vi "Parse Light IDs.vi"(8 "Error In":errorcluster, 10 "Light JSON":string="{\"1\":{\"name\": \"Hue Lamp\"},\"2\":{\"name\": \"Hue Lamp 1\"},\"3\":{\"name\": \"Hue Lamp 2\"}}") -> (0 "Error Out":errorcluster, 2 "Light IDs":i32[](array[numeric]))   [LabVIEW 2013, in "LMH-Hue.lvlib"]
uses:
  LMH-Hue.lvlib
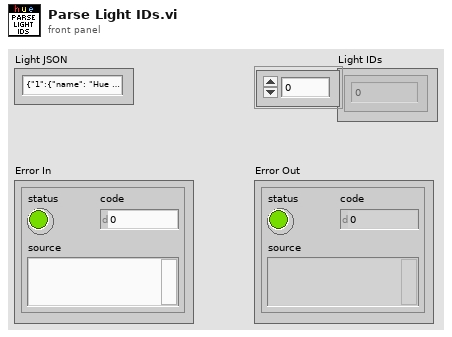
[diagram p1: front panel]
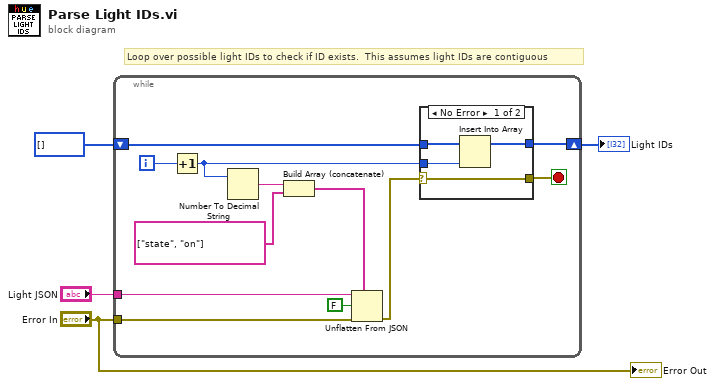
[diagram p0: block diagram]
diagram:
  # "Loop over possible light IDs to check if ID exists.  This assumes light IDs are contiguous"
  n1 = while {
    tunnel: "Light JSON" -> [w12]
    shift-right: [w9] -> w2
    shift-left: i32[] [] ("Light IDs") -> [w10]
    tunnel: "Error In" -> [w16]
    i -> [w6]
    stop <- w8 stop-if-true
    n2 = Increment(x=w6) -> (x+1=w5:i32)
    n3 = Number To Decimal String(number=w5) -> (decimal integer string=w14:string)  [unwired: 1 in]
    n4 = Build Array (concatenate)(w14, string[] ["state", "on"] ("path")) -> (w13:string[])
    n5 = Unflatten From JSON(path=w13, JSON string=w12, type and defaults=FALSE, error in (no error)=w16) -> (error out=w11:errorcluster)  [unwired: 3 in, 1 out]
    n6 = case shown="No Error" w11 {
      selector: w11 -> [w17 w21]
      tunnel: w10 -> [w20 w22]
      tunnel: w5 -> [w19 _]
      tunnel: [w18 w22] -> w9
      tunnel: [w17 w21] -> w8
      frame No Error {
        n7 = Insert Into Array(array=w20, new element=w19) -> (w18:i32[])  [unwired: 1 in]
      }
      frame Error {
      }
    }
  }
  "Light IDs" <- w2
  "Error Out" <- "Error In"
